vi "DepthFrame 1D Output Callback.vi"(4 "Data Queue Out":refnum<queue>, 5 "Event Data":cluster{"sender":refnum<k24>, "e":refnum<k24>}, 6 "Control Ref":refnum<k24>, 7 "Event Common Data":T1) -> ()   [LabVIEW 2011]
uses:
  Microsoft.Kinect
  Kinect Data Cluster.ctl
panel:
  in  "User Parameter":variant
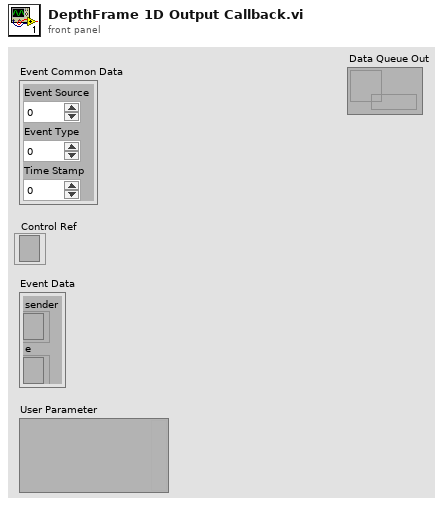
[diagram p1: front panel]
types:
  T1 = cluster{"Event Source":i32, "Event Type":u32, "Time Stamp":u32}
  T2 = typedef "Kinect Data Cluster.ctl" = cluster{"1D Depth Data":i16[], "Width":i32, "Height":i32, "Timestamp":i32}
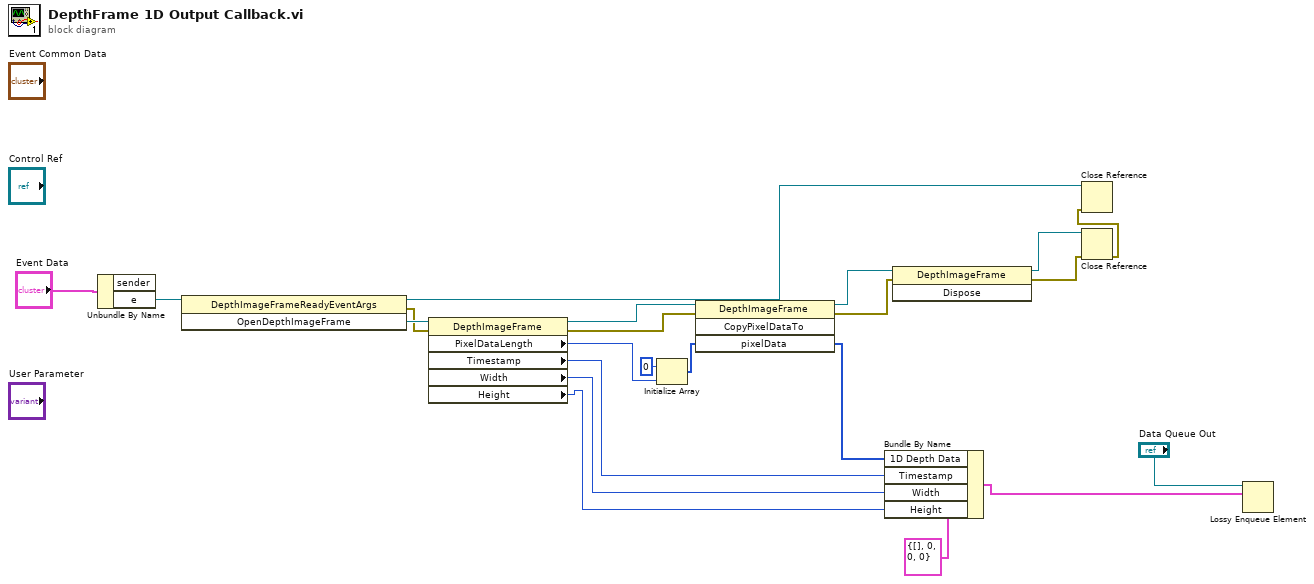
[diagram p0: block diagram]
diagram:
  n1 = Unbundle By Name("Event Data") -> ("e"=w20:refnum<k24>)  [unwired: 1 out]
  n2 = invoke class="DepthImageFrameReadyEventArgs" method="OpenDepthImageFrame"(reference=w20) -> (reference out=w18:refnum<k24>, error out=w21:errorcluster, "OpenDepthImageFrame"=w22:refnum<k24>)  [unwired: 2 in]
  n3 = property on="Property Node" class="DepthImageFrame"(reference=w22, error in=w21) -> (reference out=w13:refnum<k24>, error out=w15:errorcluster, "PixelDataLength"=w9:i32, "Timestamp"=w6:i64, "Width"=w5:i32, "Height"=w4:i32)
  n4 = Initialize Array(i16 0 ("element"), w9) -> (w10:i16[])
  n5 = invoke class="DepthImageFrame" method="CopyPixelDataTo"(reference=w13, error in=w15, "pixelData"=w10) -> (reference out=w12:refnum<k24>, error out=w14:errorcluster, "pixelData"=w2:i16[])  [unwired: 1 in, 1 out]
  n6 = Bundle By Name(cluster=T2 {"1D Depth Data"=[], "Width"=0, "Height"=0, "Timestamp"=0}, "1D Depth Data"=w2, "Timestamp"=w6, "Width"=w5, "Height"=w4) -> (w1:T2)
  n7 = invoke class="DepthImageFrame" method="Dispose"(reference=w12, error in=w14) -> (reference out=w19:refnum<k24>, error out=w17:errorcluster)  [unwired: 1 in, 1 out]
  n8 = Close Reference(reference=w19, error in (no error)=w17) -> (error out=w16:errorcluster)
  n9 = Close Reference(reference=w18, error in (no error)=w16) -> ()  [unwired: 1 out]
  n10 = Lossy Enqueue Element(queue="Data Queue Out", element=w1) -> ()  [unwired: 1 in, 4 out]
